vi "Read Method.vi"(11 "Filter in":refnum<class "Filter.lvclass">) -> (2 "Method":T1, 3 "Filter out":refnum<class "Filter.lvclass">)   [LabVIEW 2024, in "Logging.lvlib" / "Filter.lvclass"]
uses:
  Filter.lvclass
  Filter.lvclass/Filter.ctl
  Aggregation Method.ctl
  Logging.lvlib
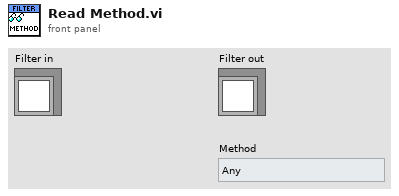
[diagram p1: front panel]
types:
  T1 = typedef "Logging.lvlib/Aggregation Method.ctl" = enum16{"Any", "Only", "All", "None"}
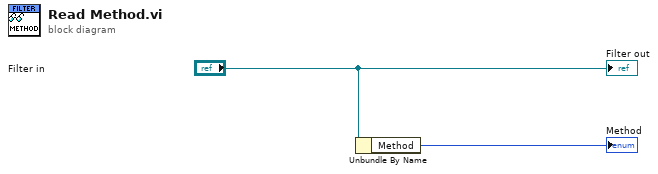
[diagram p0: block diagram]
diagram:
  n1 = Unbundle By Name("Filter in") -> ("Method"=→"Method":T1)
  "Filter out" <- "Filter in"
